vi "Disconnect.vi"(8 "error in (no error)":errorcluster, 11 "ClientBase in":refnum<class "TCP.lvclass">) -> (0 "error out":errorcluster, 3 "ClientBase out":refnum<class "TCP.lvclass">)   [LabVIEW 2020, in "TCP.lvlib" / "TCP.lvclass"]
uses:
  TCP.lvclass
  TCP.lvclass/TCP.ctl
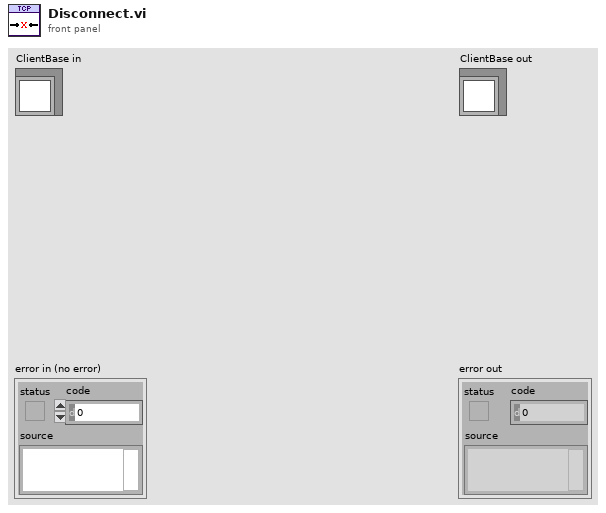
[diagram p1: front panel]
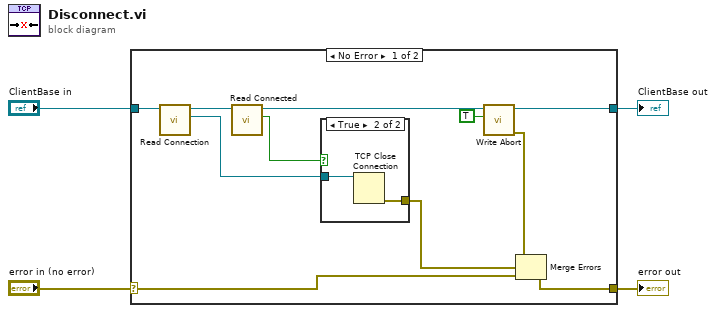
[diagram p0: block diagram]
diagram:
  n1 = case shown="No Error" "error in (no error)" {
    selector: "error in (no error)" -> [w13 w19]
    tunnel: [w14 w19] -> w3
    tunnel: [w10 w18] -> w1
    tunnel: "ClientBase in" -> [w5 w18]
    frame No Error {
      n2 = call "Read Connection.vi"("ClientBase in"=w5) -> ("Connection ID"=w9:refnum<k5>, "ClientBase out"=w7:refnum<class "TCP.lvclass">)  [unwired: 8 in, 1 out]
      n3 = call "Read Connected.vi"("ClientBase in"=w7) -> ("Connected"=w8:bool, "ClientBase out"=w6:refnum<class "TCP.lvclass">)  [unwired: 8 in, 1 out]
      n4 = case shown="True" w8 {
        tunnel: w9 -> [_ w17]
        tunnel: [_ w16] -> w15
        frame False {
        }
        frame True {
          n5 = TCP Close Connection(connection ID=w17) -> (error out=w16:errorcluster)  [unwired: 2 in, 1 out]
        }
      }
      n6 = call "Write Abort.vi"("Abort"=TRUE, "ClientBase in"=w6) -> ("error out"=w11:errorcluster, "ClientBase out"=w10:refnum<class "TCP.lvclass">)  [unwired: 8 in]
      n7 = Merge Errors(w11, w15, w13) -> (w14:errorcluster)
    }
    frame Error {
    }
  }
  "error out" <- w3
  "ClientBase out" <- w1
